vi "Cleanup Session.vi"(8 "error in":errorcluster, 11 "Plugin in":refnum<class "FFT.lvclass">) -> (0 "error out":errorcluster, 3 "Plugin out":refnum<class "FFT.lvclass">)   [LabVIEW 2024, in "FFT.lvlib" / "FFT.lvclass"]
uses:
  FFT.lvclass
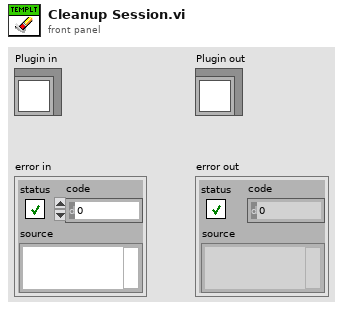
[diagram p1: front panel]
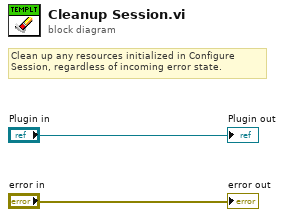
[diagram p0: block diagram]
diagram:
  # "Clean up any resources initialized in Configure Session, regardless of incoming error state."
  "error out" <- "error in"
  "Plugin out" <- "Plugin in"
